vi "Ancestor Classes.vi"(8 "error in (no error)":errorcluster, 11 "Section in":refnum<class "Section.lvclass">) -> (0 "error out":errorcluster, 1 "Ancestor Classes":string[](array[string]), 2 "Ancestor Class Pathes":path[](array[path]), 3 "Section out":refnum<class "Section.lvclass">)   [LabVIEW 2016, in "Configuration.lvlib" / "Section.lvclass"]
doc: "This VI returns array of all ancestor classes and their pathes."
uses:
  Section.lvclass
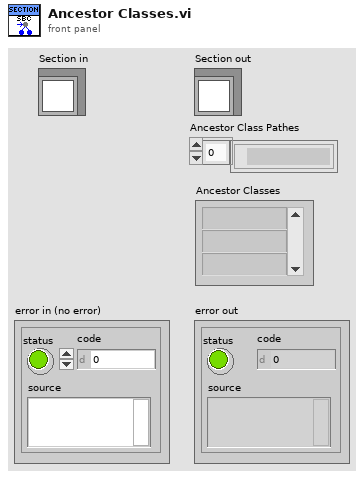
[diagram p1: front panel]
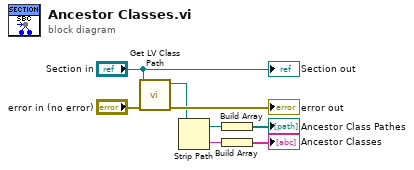
[diagram p0: block diagram]
diagram:
  n1 = call <vilib>:"Get LV Class Path.vi"("error in (no error)"="error in (no error)", "object"="Section in") -> ("error out"=→"error out":errorcluster, "class path"=w3:path)  [unwired: 8 in]
  n2 = Strip Path(path=w3) -> (stripped path=w1:path, name=w2:string)
  n3 = Build Array(w1) -> (→"Ancestor Class Pathes":path[])
  n4 = Build Array(w2) -> (→"Ancestor Classes":string[])
  "Section out" <- "Section in"
